vi "Axsun module.vi"(7 "Action":T2=enum."Clock delay", 8 "error in (no error)":errorcluster, 10 "Clock delay":dbl) -> (0 "error out":errorcluster, 2 "output cluster":T1)   [LabVIEW 2018]
uses:
  Axsun action.ctl
  serial sectioning OCT/Axsun/cluster_Axsun.ctl
  C:/Users/shuaibin/Documents/serial sectioning OCT/Axsun/AxsunOCTControl.dll
  serial sectioning OCT/Axsun/AxsunOCTControl.dll
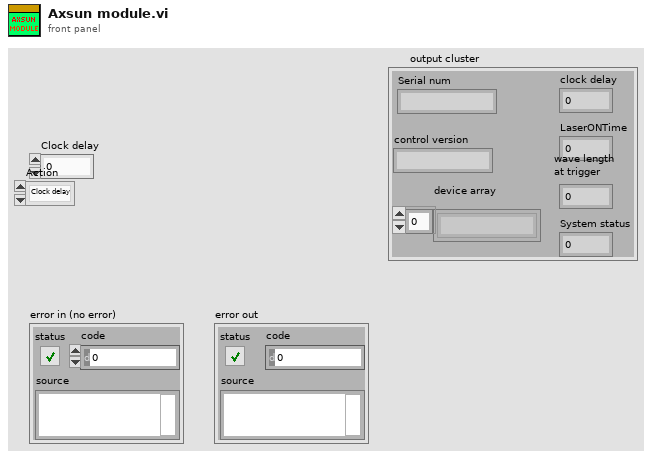
[diagram p1: front panel]
types:
  T1 = typedef "cluster_Axsun.ctl" = cluster{"device array":string[], "control version":string, "Serial num":string, "LaserONTime":i32, "wave length\nat trigger":dbl, "System status":dbl, "clock delay":u32}
  T2 = typedef "Axsun action.ctl" = enum16{"GetSystemStatus", "Clock delay", "GetLaserOnTime", "GetWaveLengthAtSweptTrigger", "Source current ON", "GetSerialNum", "GetControlVersion", "Laser ON", "Laser OFF", "Source current OFF", "Get laser handle", "Start Network Control Interface", "stop", "Create handle"}
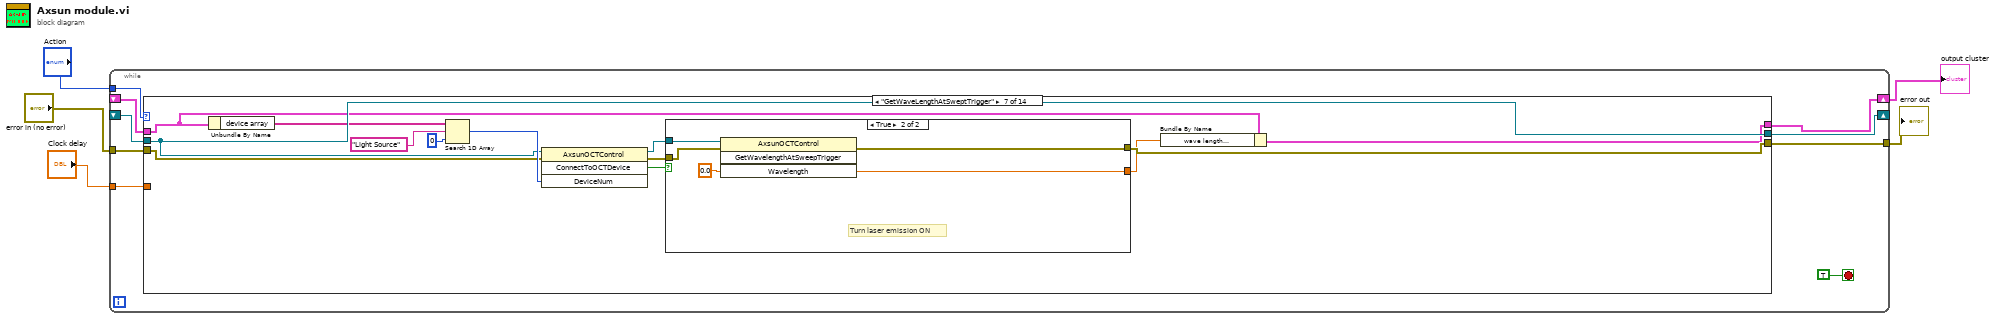
[diagram p0: block diagram]
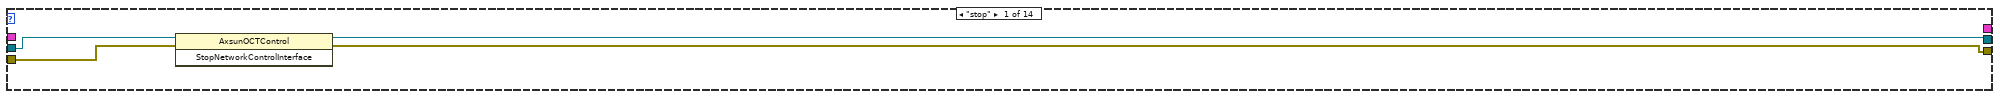
[diagram p2: hidden frame]
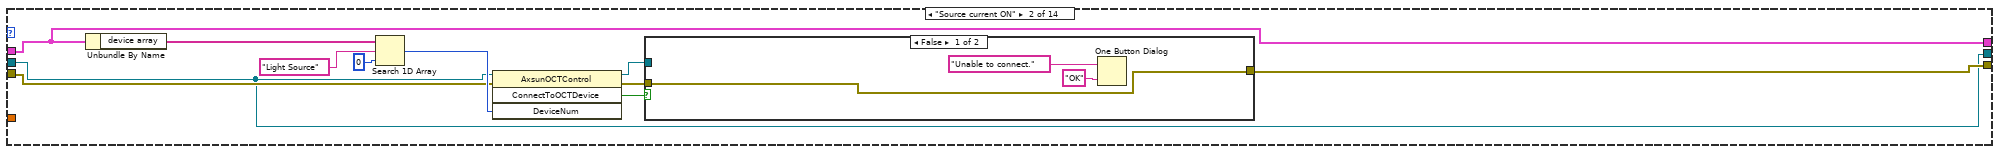
[diagram p3: hidden frame]
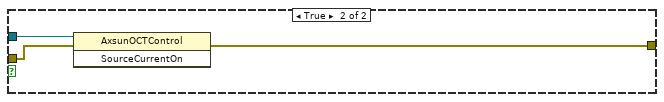
[diagram p4: hidden frame]
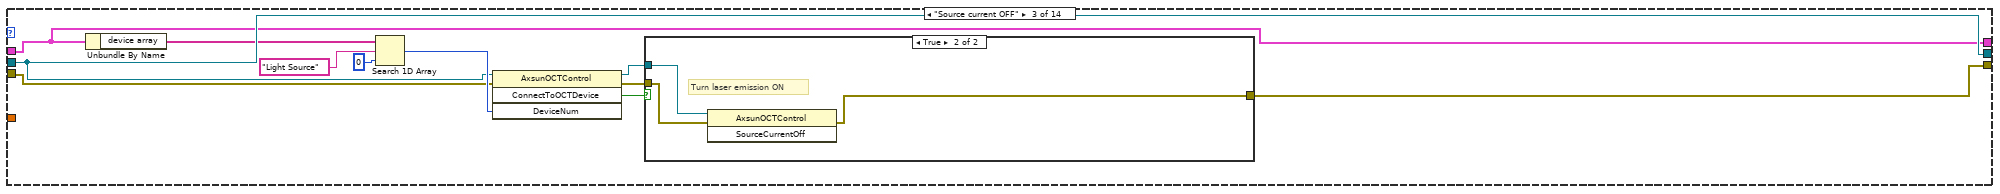
[diagram p5: hidden frame]
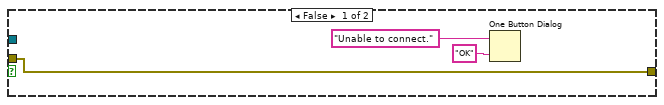
[diagram p6: hidden frame]
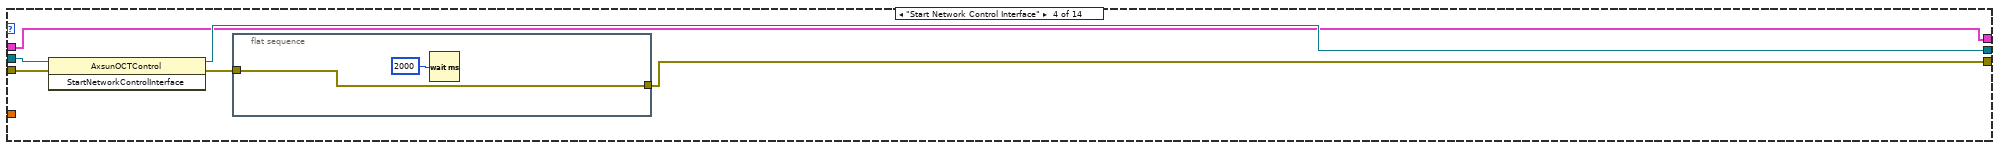
[diagram p7: hidden frame]
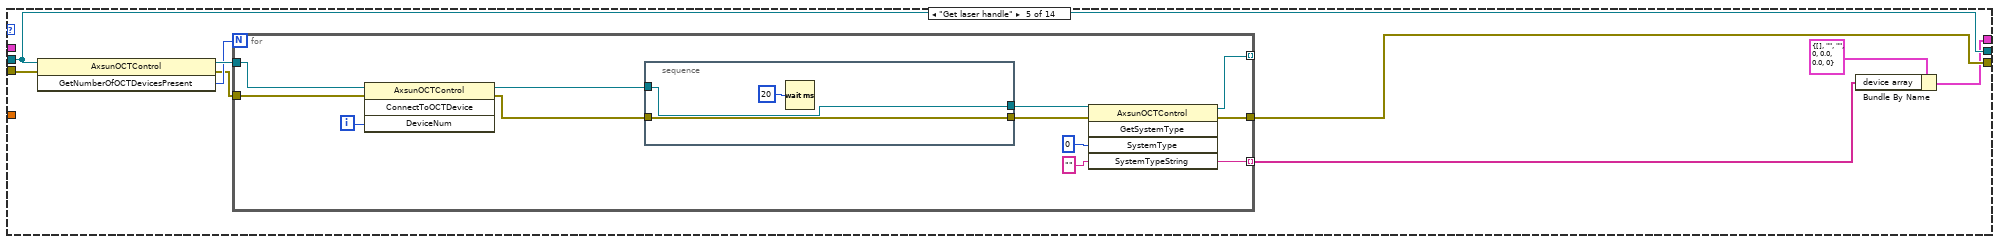
[diagram p8: hidden frame]
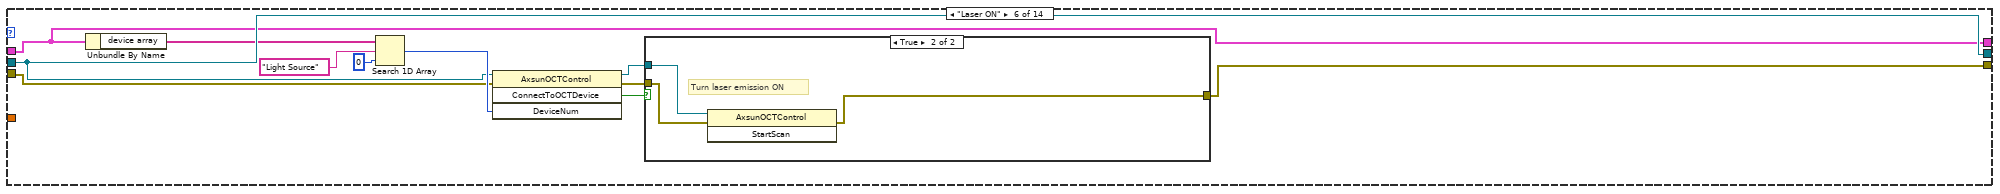
[diagram p9: hidden frame]
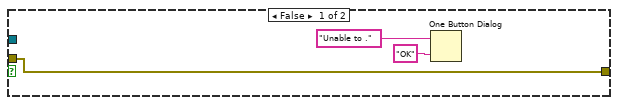
[diagram p10: hidden frame]
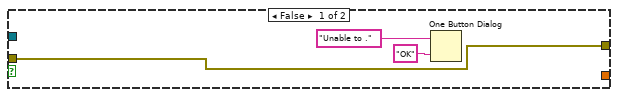
[diagram p11: hidden frame]
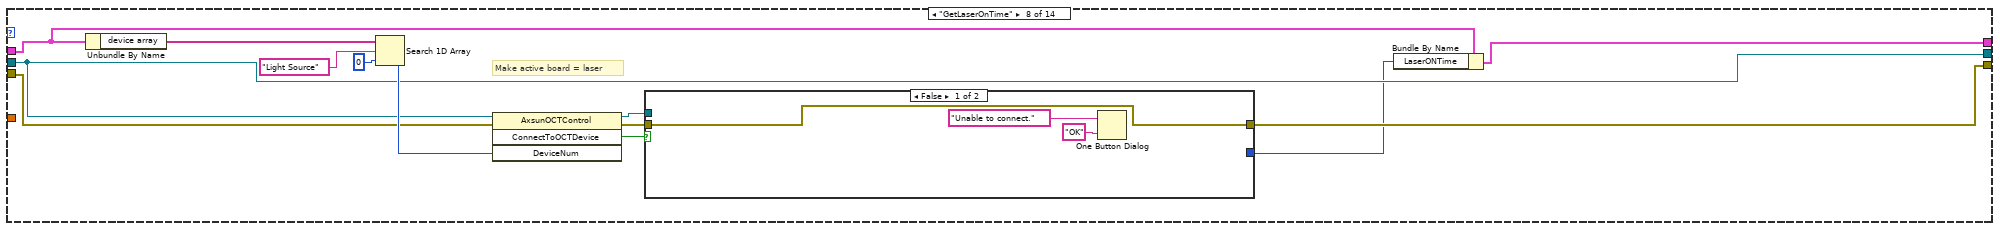
[diagram p12: hidden frame]
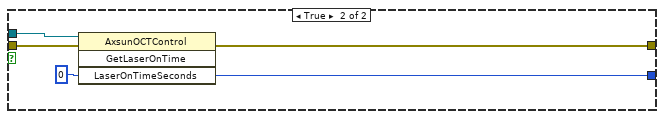
[diagram p13: hidden frame]
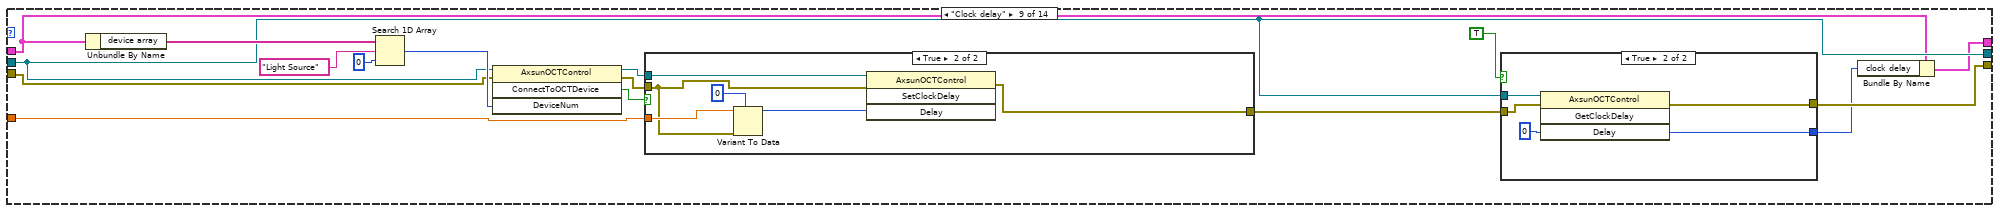
[diagram p14: hidden frame]
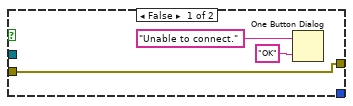
[diagram p15: hidden frame]
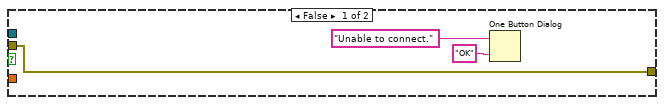
[diagram p16: hidden frame]
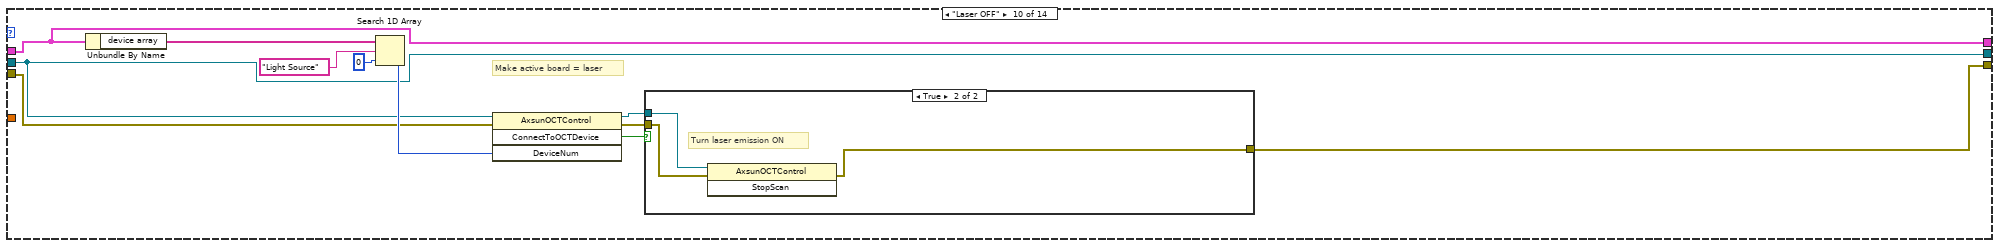
[diagram p17: hidden frame]
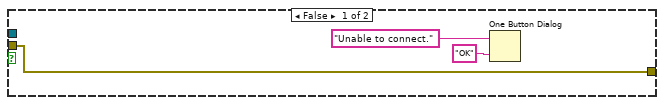
[diagram p18: hidden frame]
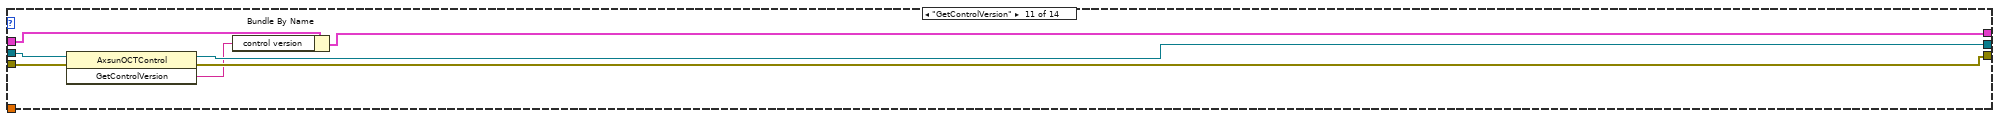
[diagram p19: hidden frame]
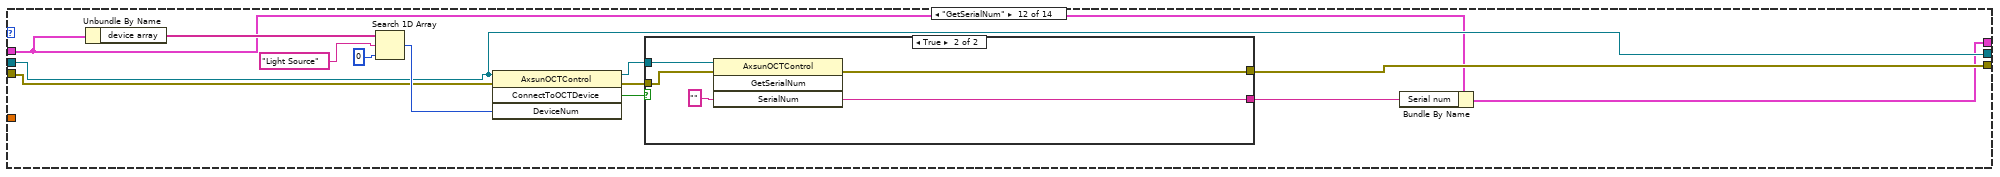
[diagram p20: hidden frame]
diagram:
  n1 = while {
    shift-right: [w13] -> _
    shift-left: _ -> [w12]
    tunnel: "error in (no error)" -> [w14]
    shift-right: [w9] -> w1
    shift-left: _ -> [w11]
    tunnel: [w10] -> w3
    tunnel: "Action" -> [w8]
    tunnel: "Clock delay" -> [w7]
    stop <- TRUE stop-if-true
    n2 = case shown="\"GetWaveLengthAtSweptTrigger\"" w8 {
      tunnel: w14 -> [w17 w23 w39 w57 w69 w89 w107 w129 w152 w181 w199 w206 w227 _]
      tunnel: [w16 w21 w38 w54 w64 w87 w108 w127 w149 w179 w197 w207 _ w246] -> w13
      tunnel: w12 -> [w18 w21 w38 w58 w64 w87 w108 w127 w149 w179 w200 w207 w228 _]
      tunnel: [w15 w22 w40 w55 w65 w88 w106 w128 w148 w180 w198 w205 w226 w245] -> w10
      tunnel: [_ w20 w37 w53 w62 w86 w103 w124 w146 w178 w195 w201 w222 w244] -> w9
      tunnel: w11 -> [_ w20 w37 w53 _ w86 w104 w125 w147 w178 w196 w203 w224 w244]
      tunnel: w7 -> [_ _ _ _ _ _ _ _ w144 _ _ _ _ _]
      frame "stop" {
        n3 = invoke class="AxsunOCTControl" method="StopNetworkControlInterface"(reference=w18, error in=w17) -> (reference out=w16:refnum<k24>, error out=w15:errorcluster)  [unwired: 1 in, 1 out]
      }
      frame "Source current ON" {
        n4 = Unbundle By Name(w20) -> ("device array"=w19:string[])
        n5 = Search 1D Array(1D array=w19, element="Light Source", start index (0)=0) -> (index of element=w27:i32)
        n6 = invoke class="AxsunOCTControl" method="ConnectToOCTDevice"(reference=w21, error in=w23, "DeviceNum"=w27) -> (reference out=w26:refnum<k24>, error out=w25:errorcluster, "ConnectToOCTDevice"=w24:bool)  [unwired: 1 in, 1 out]
        n7 = case shown="False" w24 {
          tunnel: w26 -> [_ w35]
          tunnel: w25 -> [w32 w34]
          tunnel: [w32 w33] -> w22
          frame False {
            n8 = One Button Dialog(message="Unable to connect.", button name ("OK")="OK") -> ()  [unwired: 1 out]
          }
          frame True {
            n9 = invoke class="AxsunOCTControl" method="SourceCurrentOn"(reference=w35, error in=w34) -> (error out=w33:errorcluster)  [unwired: 1 in, 2 out]
          }
        }
      }
      frame "Source current OFF" {
        n10 = Unbundle By Name(w37) -> ("device array"=w36:string[])
        n11 = Search 1D Array(1D array=w36, element="Light Source", start index (0)=0) -> (index of element=w44:i32)
        n12 = invoke class="AxsunOCTControl" method="ConnectToOCTDevice"(reference=w38, error in=w39, "DeviceNum"=w44) -> (reference out=w43:refnum<k24>, error out=w42:errorcluster, "ConnectToOCTDevice"=w41:bool)  [unwired: 1 in, 1 out]
        n13 = case shown="True" w41 {
          tunnel: w43 -> [_ w52]
          tunnel: w42 -> [w49 w51]
          tunnel: [w49 w50] -> w40
          frame False {
            n14 = One Button Dialog(message="Unable to connect.", button name ("OK")="OK") -> ()  [unwired: 1 out]
          }
          frame True {
            # "Turn laser emission ON"
            n15 = invoke class="AxsunOCTControl" method="SourceCurrentOff"(reference=w52, error in=w51) -> (error out=w50:errorcluster)  [unwired: 1 in, 2 out]
          }
        }
      }
      frame "Start Network Control Interface" {
        n16 = invoke class="AxsunOCTControl" method="StartNetworkControlInterface"(reference=w58, error in=w57) -> (reference out=w54:refnum<k24>, error out=w56:errorcluster)  [unwired: 1 in, 1 out]
        n17 = flat-sequence {
          tunnel: w56 -> [w59]
          tunnel: [w59] -> w55
          frame #0 {
            n18 = Wait (ms)(milliseconds to wait=2000) -> ()  [unwired: 1 out]
          }
        }
      }
      frame "Get laser handle" {
        n19 = invoke class="AxsunOCTControl" method="GetNumberOfOCTDevicesPresent"(reference=w64, error in=w69) -> (reference out=w68:refnum<k24>, error out=w66:errorcluster, "GetNumberOfOCTDevicesPresent"=w67:i32)  [unwired: 1 in]
        n20 = for {
          N: w67 -> [_]
          tunnel: w68 -> [w75]
          tunnel: w66 -> [w74]
          tunnel: [w70] -> w61 mode=indexing
          tunnel: [w72] -> w65
          tunnel: [w71] -> _ mode=indexing
          i -> [w73]
          n21 = invoke class="AxsunOCTControl" method="ConnectToOCTDevice"(reference=w75, error in=w74, "DeviceNum"=w73) -> (reference out=w79:refnum<k24>, error out=w78:errorcluster)  [unwired: 1 in, 2 out]
          n22 = stacked-sequence {
            tunnel: w79 -> [w84]
            tunnel: [w84] -> w77
            tunnel: w78 -> [w83]
            tunnel: [w83] -> w76
            frame #0 {
              n23 = Wait (ms)(milliseconds to wait=u32 20) -> ()  [unwired: 1 out]
            }
          }
          n24 = invoke class="AxsunOCTControl" method="GetSystemType"(reference=w77, error in=w76, "SystemType"=u32 0, "SystemTypeString"="") -> (reference out=w71:refnum<k24>, error out=w72:errorcluster, "SystemTypeString"=w70:string)  [unwired: 1 in, 2 out]
        }
        n25 = Bundle By Name(cluster=T1 {"device array"=[], "control version"="", "Serial num"="", "LaserONTime"=0, "wave length\nat trigger"=0.0, "System status"=0.0, "clock delay"=0} ("output cluster"), "device array"=w61) -> (w62:T1)
      }
      frame "Laser ON" {
        n26 = Unbundle By Name(w86) -> ("device array"=w85:string[])
        n27 = Search 1D Array(1D array=w85, element="Light Source", start index (0)=0) -> (index of element=w93:i32)
        n28 = invoke class="AxsunOCTControl" method="ConnectToOCTDevice"(reference=w87, error in=w89, "DeviceNum"=w93) -> (reference out=w92:refnum<k24>, error out=w91:errorcluster, "ConnectToOCTDevice"=w90:bool)  [unwired: 1 in, 1 out]
        n29 = case shown="True" w90 {
          tunnel: w92 -> [_ w101]
          tunnel: w91 -> [w98 w100]
          tunnel: [w98 w99] -> w88
          frame False {
            n30 = One Button Dialog(message="Unable to .", button name ("OK")="OK") -> ()  [unwired: 1 out]
          }
          frame True {
            # "Turn laser emission ON"
            n31 = invoke class="AxsunOCTControl" method="StartScan"(reference=w101, error in=w100) -> (error out=w99:errorcluster)  [unwired: 1 in, 2 out]
          }
        }
      }
      frame "GetWaveLengthAtSweptTrigger" {
        n32 = Unbundle By Name(w104) -> ("device array"=w105:string[])
        n33 = Search 1D Array(1D array=w105, element="Light Source", start index (0)=0) -> (index of element=w112:i32)
        n34 = invoke class="AxsunOCTControl" method="ConnectToOCTDevice"(reference=w108, error in=w107, "DeviceNum"=w112) -> (reference out=w111:refnum<k24>, error out=w110:errorcluster, "ConnectToOCTDevice"=w109:bool)  [unwired: 1 in, 1 out]
        n35 = case shown="True" w109 {
          tunnel: w111 -> [_ w122]
          tunnel: w110 -> [w117 w121]
          tunnel: [w117 w120] -> w106
          tunnel: [_ w118] -> w102
          frame False {
            n36 = One Button Dialog(message="Unable to .", button name ("OK")="OK") -> ()  [unwired: 1 out]
          }
          frame True {
            # "Turn laser emission ON"
            n37 = invoke class="AxsunOCTControl" method="GetWavelengthAtSweepTrigger"(reference=w122, error in=w121, "Wavelength"=0.0) -> (error out=w120:errorcluster, "Wavelength"=w118:dbl)  [unwired: 1 in, 2 out]
          }
        }
        n38 = Bundle By Name(cluster=w104, "wave length\nat trigger"=w102) -> (w103:T1)
      }
      frame "GetLaserOnTime" {
        # "Make active board = laser"
        n39 = Unbundle By Name(w125) -> ("device array"=w126:string[])
        n40 = Search 1D Array(1D array=w126, element="Light Source", start index (0)=0) -> (index of element=w135:i32)
        n41 = invoke class="AxsunOCTControl" method="ConnectToOCTDevice"(reference=w127, error in=w129, "DeviceNum"=w135) -> (reference out=w131:refnum<k24>, error out=w132:errorcluster, "ConnectToOCTDevice"=w130:bool)  [unwired: 1 in, 1 out]
        n42 = case shown="False" w130 {
          tunnel: w132 -> [w138 w142]
          tunnel: w131 -> [_ w143]
          tunnel: [w138 w141] -> w128
          tunnel: [_ w139] -> w123
          frame False {
            n43 = One Button Dialog(message="Unable to connect.", button name ("OK")="OK") -> ()  [unwired: 1 out]
          }
          frame True {
            n44 = invoke class="AxsunOCTControl" method="GetLaserOnTime"(reference=w143, error in=w142, "LaserOnTimeSeconds"=u32 0) -> (error out=w141:errorcluster, "LaserOnTimeSeconds"=w139:u32)  [unwired: 1 in, 2 out]
          }
        }
        n45 = Bundle By Name(cluster=w125, "LaserONTime"=w123) -> (w124:T1)
      }
      frame "Clock delay" {
        n46 = Unbundle By Name(w147) -> ("device array"=w153:string[])
        n47 = Search 1D Array(1D array=w153, element="Light Source", start index (0)=0) -> (index of element=w157:i32)
        n48 = invoke class="AxsunOCTControl" method="ConnectToOCTDevice"(reference=w149, error in=w152, "DeviceNum"=w157) -> (reference out=w156:refnum<k24>, error out=w155:errorcluster, "ConnectToOCTDevice"=w154:bool)  [unwired: 1 in, 1 out]
        n49 = case shown="True" w154 {
          tunnel: w156 -> [_ w176]
          tunnel: w155 -> [w170 w172]
          tunnel: [w170 w171] -> w151
          tunnel: w144 -> [_ w175]
          frame False {
            n50 = One Button Dialog(message="Unable to connect.", button name ("OK")="OK") -> ()  [unwired: 1 out]
          }
          frame True {
            n51 = Variant To Data(error in=w172, type=u32 0 ("Delay"), Variant=w175) -> (data=w173:u32)  [unwired: 1 out]
            n52 = invoke class="AxsunOCTControl" method="SetClockDelay"(reference=w176, error in=w172, "Delay"=w173) -> (error out=w171:errorcluster)  [unwired: 1 in, 3 out]
          }
        }
        n53 = case shown="True" TRUE {
          tunnel: w151 -> [w162 w166]
          tunnel: w149 -> [_ w167]
          tunnel: [w162 w165] -> w148
          tunnel: [_ w163] -> w145
          frame False {
            n54 = One Button Dialog(message="Unable to connect.", button name ("OK")="OK") -> ()  [unwired: 1 out]
          }
          frame True {
            n55 = invoke class="AxsunOCTControl" method="GetClockDelay"(reference=w167, error in=w166, "Delay"=u32 0) -> (error out=w165:errorcluster, "Delay"=w163:u32)  [unwired: 1 in, 2 out]
          }
        }
        n56 = Bundle By Name(cluster=w147, "clock delay"=w145) -> (w146:T1)
      }
      frame "Laser OFF" {
        # "Make active board = laser"
        n57 = Unbundle By Name(w178) -> ("device array"=w177:string[])
        n58 = Search 1D Array(1D array=w177, element="Light Source", start index (0)=0) -> (index of element=w185:i32)
        n59 = invoke class="AxsunOCTControl" method="ConnectToOCTDevice"(reference=w179, error in=w181, "DeviceNum"=w185) -> (reference out=w184:refnum<k24>, error out=w183:errorcluster, "ConnectToOCTDevice"=w182:bool)  [unwired: 1 in, 1 out]
        n60 = case shown="True" w182 {
          tunnel: w184 -> [_ w193]
          tunnel: w183 -> [w190 w192]
          tunnel: [w190 w191] -> w180
          frame False {
            n61 = One Button Dialog(message="Unable to connect.", button name ("OK")="OK") -> ()  [unwired: 1 out]
          }
          frame True {
            # "Turn laser emission ON"
            n62 = invoke class="AxsunOCTControl" method="StopScan"(reference=w193, error in=w192) -> (error out=w191:errorcluster)  [unwired: 1 in, 2 out]
          }
        }
      }
      frame "GetControlVersion" {
        n63 = invoke class="AxsunOCTControl" method="GetControlVersion"(reference=w200, error in=w199) -> (reference out=w197:refnum<k24>, error out=w198:errorcluster, "GetControlVersion"=w194:string)  [unwired: 1 in]
        n64 = Bundle By Name(cluster=w196, "control version"=w194) -> (w195:T1)
      }
      frame "GetSerialNum" {
        n65 = Unbundle By Name(w203) -> ("device array"=w204:string[])
        n66 = Search 1D Array(1D array=w204, element="Light Source", start index (0)=0) -> (index of element=w211:i32)
        n67 = invoke class="AxsunOCTControl" method="ConnectToOCTDevice"(reference=w207, error in=w206, "DeviceNum"=w211) -> (reference out=w210:refnum<k24>, error out=w209:errorcluster, "ConnectToOCTDevice"=w208:bool)  [unwired: 1 in, 1 out]
        n68 = case shown="True" w208 {
          tunnel: w210 -> [_ w221]
          tunnel: w209 -> [w216 w220]
          tunnel: [w216 w219] -> w205
          tunnel: [_ w217] -> w202
          frame False {
            n69 = One Button Dialog(message="Unable to connect.", button name ("OK")="OK") -> ()  [unwired: 1 out]
          }
          frame True {
            n70 = invoke class="AxsunOCTControl" method="GetSerialNum"(reference=w221, error in=w220, "SerialNum"="") -> (error out=w219:errorcluster, "SerialNum"=w217:string)  [unwired: 1 in, 2 out]
          }
        }
        n71 = Bundle By Name(cluster=w203, "Serial num"=w202) -> (w201:T1)
      }
      frame "GetSystemStatus" {
        # "Make active board = laser"
        n72 = Unbundle By Name(w224) -> ("device array"=w225:string[])
        n73 = Search 1D Array(1D array=w225, element="Light Source", start index (0)=0) -> (index of element=w234:i32)
        n74 = invoke class="AxsunOCTControl" method="ConnectToOCTDevice"(reference=w228, error in=w227, "DeviceNum"=w234) -> (reference out=w229:refnum<k24>, error out=w230:errorcluster, "ConnectToOCTDevice"=w231:bool)  [unwired: 1 in, 1 out]
        n75 = case shown="True" w231 {
          tunnel: w230 -> [w237 w242]
          tunnel: w229 -> [_ w243]
          tunnel: [w237 w239] -> w226
          tunnel: [_ w238] -> w223
          frame False {
            n76 = One Button Dialog(message="Unable to connect.", button name ("OK")="OK") -> ()  [unwired: 1 out]
          }
          frame True {
            n77 = invoke class="AxsunOCTControl" method="GetSystemStatus"(reference=w243, error in=w242, "StatusArray"=u32[] [], "StatusWordsReturned"=u32 0) -> (error out=w239:errorcluster, "StatusWordsReturned"=w238:u32)  [unwired: 1 in, 3 out]
          }
        }
        n78 = Bundle By Name(cluster=w224, "System status"=w223) -> (w222:T1)
      }
      frame "Create handle" {
        n79 = constructor class="AxsunOCTControl"() -> (reference out=w246:refnum<k24>, error out=w245:errorcluster)  [unwired: 3 in, 1 out]
      }
    }
  }
  "error out" <- w3
  "output cluster" <- w1
